vi "ClimberTest.vi"(10 "progress":string, 11 "progressText":string) -> (3 "endTestText":string)   [LabVIEW 2012]
uses:
  ClimberLimitSwitches.ctl
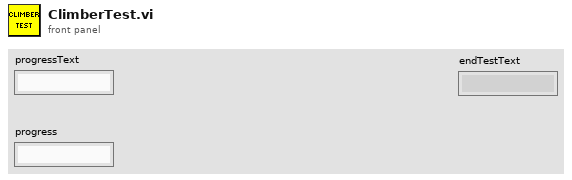
[diagram p1: front panel]
types:
  T1 = typedef "ClimberLimitSwitches.ctl" = enum16{"Off", "Bottom", "1", "2", "3", "4", "Top"}
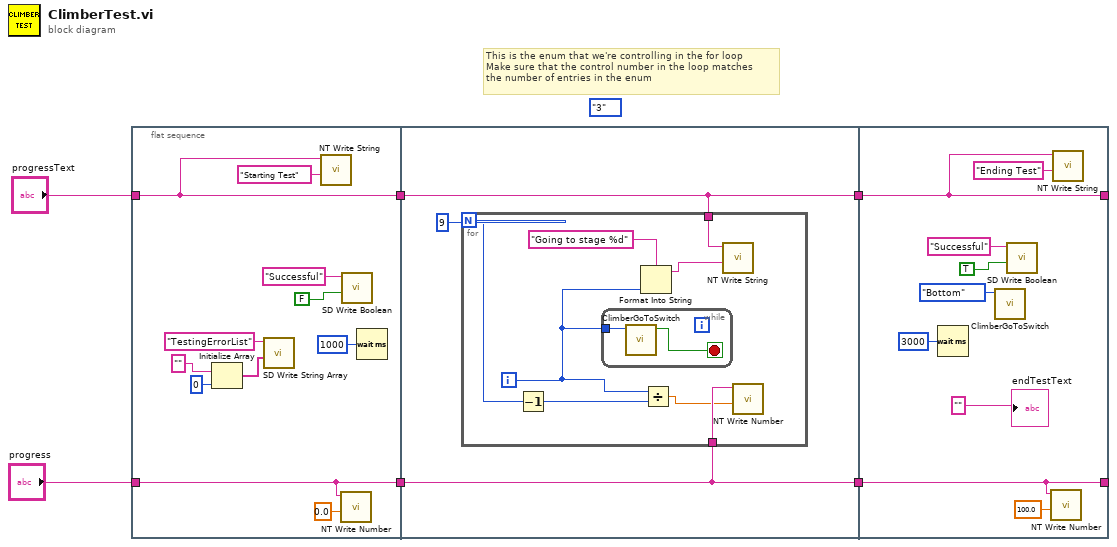
[diagram p0: block diagram]
diagram:
  (unwired) ClimberLimitSwitches."3" ("Switch")
  # "This is the enum that we're controlling in the for loop\nMake sure that the control number in the loop matches\nthe number of entries in the enum"
  n1 = flat-sequence {
    tunnel: "progressText" -> [w9]
    tunnel: "progress" -> [w8]
    tunnel: [w9] -> w4
    tunnel: [w8] -> w3
    tunnel: w4 -> [w19]
    tunnel: w3 -> [w18]
    tunnel: [w19] -> w2
    tunnel: [w18] -> w1
    tunnel: [w37] -> _
    tunnel: [w38] -> _
    tunnel: w2 -> [w38]
    tunnel: w1 -> [w37]
    frame #0 {
      n2 = Initialize Array("", 0 ("dimension size")) -> (w12:string[])
      n3 = call <vilib>:"SD Write String Array.vi"("String Array"=w12, "Name"="TestingErrorList") -> ()  [unwired: 8 in, 2 out]
      n4 = call <vilib>:"NT Write String.vi"("String"="Starting Test", "Name"=w9) -> ()  [unwired: 9 in, 1 out]
      n5 = call <vilib>:"NT Write Number.vi"("Numeric"=0.0, "Name"=w8) -> ()  [unwired: 9 in, 1 out]
      n6 = call <vilib>:"SD Write Boolean.vi"("Boolean"=FALSE, "Name"="Successful") -> ()  [unwired: 8 in, 2 out]
      n7 = Wait (ms)(milliseconds to wait=u32 1000) -> ()  [unwired: 1 out]
    }
    frame #1 {
      n8 = for {
        N: 9 -> [w23]
        tunnel: w19 -> [w26]
        tunnel: w18 -> [w25]
        i -> [w21]
        n9 = Decrement(x=w23) -> (x-1=w22:i32)
        n10 = while {
          tunnel: w21 -> [w29]
          stop <- w30 stop-if-true
          n11 = call "ClimberGoToSwitch.vi"("TargetSwitch"=w29) -> ("Done"=w30:bool)  [unwired: 10 in]
        }
        n12 = Format Into String(format string="Going to stage %d", w21) -> (resulting string=w27:string)  [unwired: 2 in, 1 out]
        n13 = Divide(x=w21, y=w22) -> (x/y=w24:dbl)
        n14 = call <vilib>:"NT Write String.vi"("String"=w27, "Name"=w26) -> ()  [unwired: 9 in, 1 out]
        n15 = call <vilib>:"NT Write Number.vi"("Numeric"=w24, "Name"=w25) -> ()  [unwired: 9 in, 1 out]
      }
    }
    frame #2 {
      n16 = Wait (ms)(milliseconds to wait=u32 3000) -> ()  [unwired: 1 out]
      n17 = call "ClimberGoToSwitch.vi"("TargetSwitch"=ClimberLimitSwitches."Bottom") -> ()  [unwired: 10 in, 1 out]
      n18 = call <vilib>:"SD Write Boolean.vi"("Boolean"=TRUE, "Name"="Successful") -> ()  [unwired: 8 in, 2 out]
      n19 = call <vilib>:"NT Write Number.vi"("Numeric"=100.0, "Name"=w37) -> ()  [unwired: 9 in, 1 out]
      n20 = call <vilib>:"NT Write String.vi"("String"="Ending Test", "Name"=w38) -> ()  [unwired: 9 in, 1 out]
      "endTestText" <- "" ("endTestText")
    }
  }
